vi "niRFUtil RFHS Math Divide Array by Value CSG.vi"(0 "data in":csg[](array[numeric]), 2 "RFHS?":bool=TRUE, 5 "divisor in":csg, 7 "result in":csg[](array[numeric]), 11 "error in":errorcluster) -> (4 "result out":csg[](array[numeric]), 15 "error out":errorcluster)   [LabVIEW 2015, in "niRFUtil.lvlib"]
uses:
  niRFUtil.lvlib
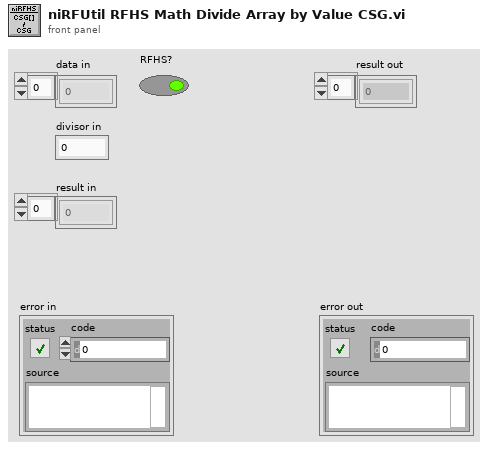
[diagram p1: front panel]
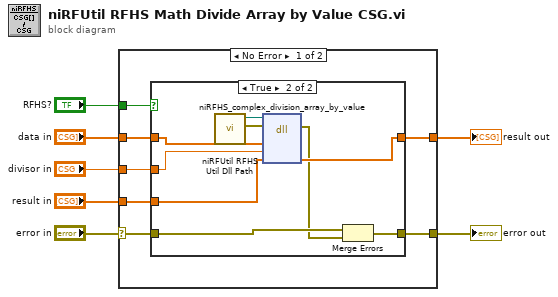
[diagram p0: block diagram]
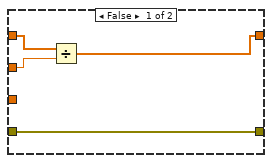
[diagram p2: hidden frame]
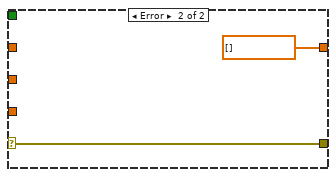
[diagram p3: hidden frame]
diagram:
  n1 = case shown="No Error" "error in" {
    selector: "error in" -> [w10 w29]
    tunnel: "RFHS?" -> [w14 _]
    tunnel: "data in" -> [w13 _]
    tunnel: "divisor in" -> [w12 _]
    tunnel: [w11 csg[] [] ("result")] -> w5
    tunnel: [w9 w29] -> w3
    tunnel: "result in" -> [w8 _]
    frame No Error {
      n2 = case shown="True" w14 {
        tunnel: w13 -> [w18 w27]
        tunnel: w12 -> [w17 w26]
        tunnel: [w16 w25] -> w11
        tunnel: w10 -> [w15 w22]
        tunnel: [w15 w20] -> w9
        tunnel: w8 -> [_ w19]
        frame False {
          n3 = Divide(x=w18, y=w17) -> (x/y=w16:csg[])
        }
        frame True {
          n4 = call "niRFUtil RFHS Util Dll Path.vi"() -> ("error out"=w24:errorcluster, "Path"=w23:path)  [unwired: 7 in, 3 out]
          n5 = dll-call lib="R:/niRFHS.dll" fn="niRFHS_complex_division_array_by_value"(path in=w23, error in=w24, "data"=w27, "divisor"=w26, "result"=w19) -> (error out=w21:errorcluster, "result"=w25:csg[])  [unwired: 4 in, 1 out]
          n6 = Merge Errors(w22, w21) -> (w20:errorcluster)
        }
      }
    }
    frame Error {
    }
  }
  "result out" <- w5
  "error out" <- w3
